vi "promptFileDialogIfNecessary.vi"(8 "error in":errorcluster, 11 "File Path":path) -> (0 "error out":errorcluster, 3 "selected path":path)   [LabVIEW 2017, in "Document API.lvlib" / "Document API.lvclass"]
doc: "Ensures the <b>File Path</b> is valid. \n\nNotes:\n - If file path is empty (default) or is <Not A Path> or is a directory, the VI displays a dialog box from which you can select a file. Error 43 occurs if you cancel the dialog box."
uses:
  Document API.lvclass
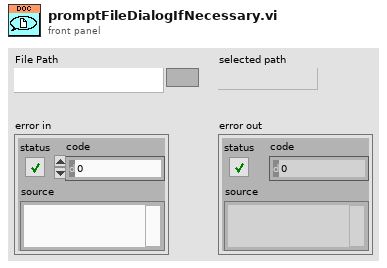
[diagram p1: front panel]
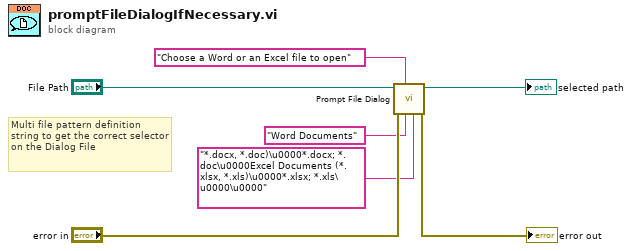
[diagram p0: block diagram]
diagram:
  # "Multi file pattern definition string to get the correct selector on the Dialog File"
  n1 = call "Prompt File Dialog.vi"("pattern (all files)"="*.docx, *.doc)\u0000*.docx; *.doc\u0000Excel Documents (*.xlsx, *.xls)\u0000*.xlsx; *.xls\u0000\u0000", "pattern label"="Word Documents", "prompt"="Choose a Word or an Excel file to open", "error in"="error in", "File Path"="File Path") -> ("error out"=→"error out":errorcluster, "selected path"=→"selected path":path)  [unwired: 5 in]
